vi "to_json.vi"(8 "error in":errorcluster, 11 "topic in":refnum<class "topic.lvclass">) -> (0 "error out":errorcluster, 2 "json":string, 3 "topic out":refnum<class "topic.lvclass">, 4 "Not Default":bool)   [LabVIEW 2020, in "nominal types.lvlib" / "channelFilter.lvlib" / "topic.lvclass"]
uses:
  topic.lvclass
  topic.lvclass/topic.ctl
  f4ac0dc0-1a1f-4287-8c6a-adac34cc9fd8.vi
  <vilib>/JDP Science/JSONtext/Variant to JSON Text.vi
  <vilib>/JDP Science/JSONtext/LVClass Serializer/JSONtext LVClass Serializer.lvclass
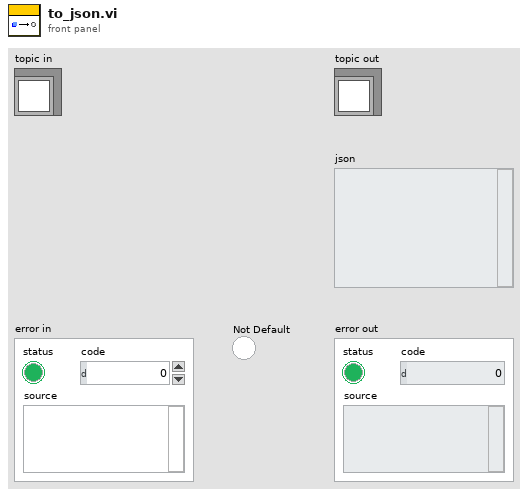
[diagram p1: front panel]
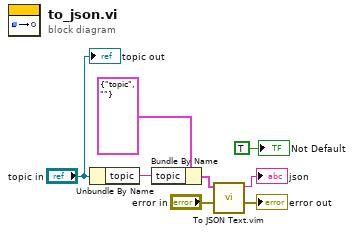
[diagram p0: block diagram]
diagram:
  n1 = Unbundle By Name("topic in") -> ("topic"=w5:string)
  n2 = Bundle By Name(cluster=cluster{"type":string, "topic":string} {"type"="topic", "topic"=""}, "topic"=w5) -> (w7:cluster{"type":string, "topic":string})
  n3 = call "To JSON Text.vim"("error in (no error)"="error in", "Anything"=w7) -> ("error out"=→"error out":errorcluster, "<JSON>"=→"json":string)  [unwired: 8 in]
  "topic out" <- "topic in"
  "Not Default" <- TRUE ("Not Default")
